vi "Multiple Connections - Server - TCP.vi"() -> ()   [LabVIEW 2011]
doc: "Demonstrates how to establish multiple connections and place them in a queue to be serviced. As connections are made, it sends the current date and time via TCP to all Client VIs that connect to it.\n\nThis VI has two parts -- a loop that listens for each client to connect, and a loop that sends the date and time to each connection in the queue.\n\n<B>Note:</B> Use this VI with Multiple Connections - Client 1.vi and Multiple Connections - Client 2.vi."
panel:
  out "Internal":i32
  out "External":i32
  in  "Port 1":u16=6341
  in  "Port 2":u16=6342
  out "#2 Connections":i32
  out "#1 Connections":i32
  in  "stop":bool
  # "Internal Network"
  # "External Network"
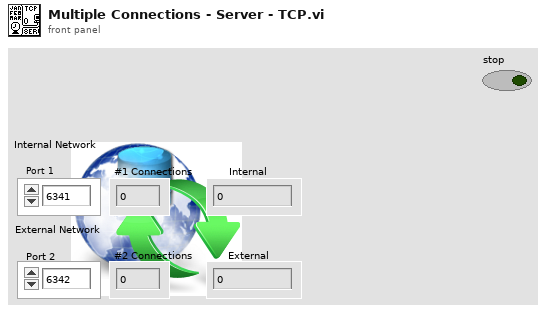
[diagram p1: front panel]
types:
  T1 = enum16{"Obtain", "Enqueue", "Dequeue", "Release"}
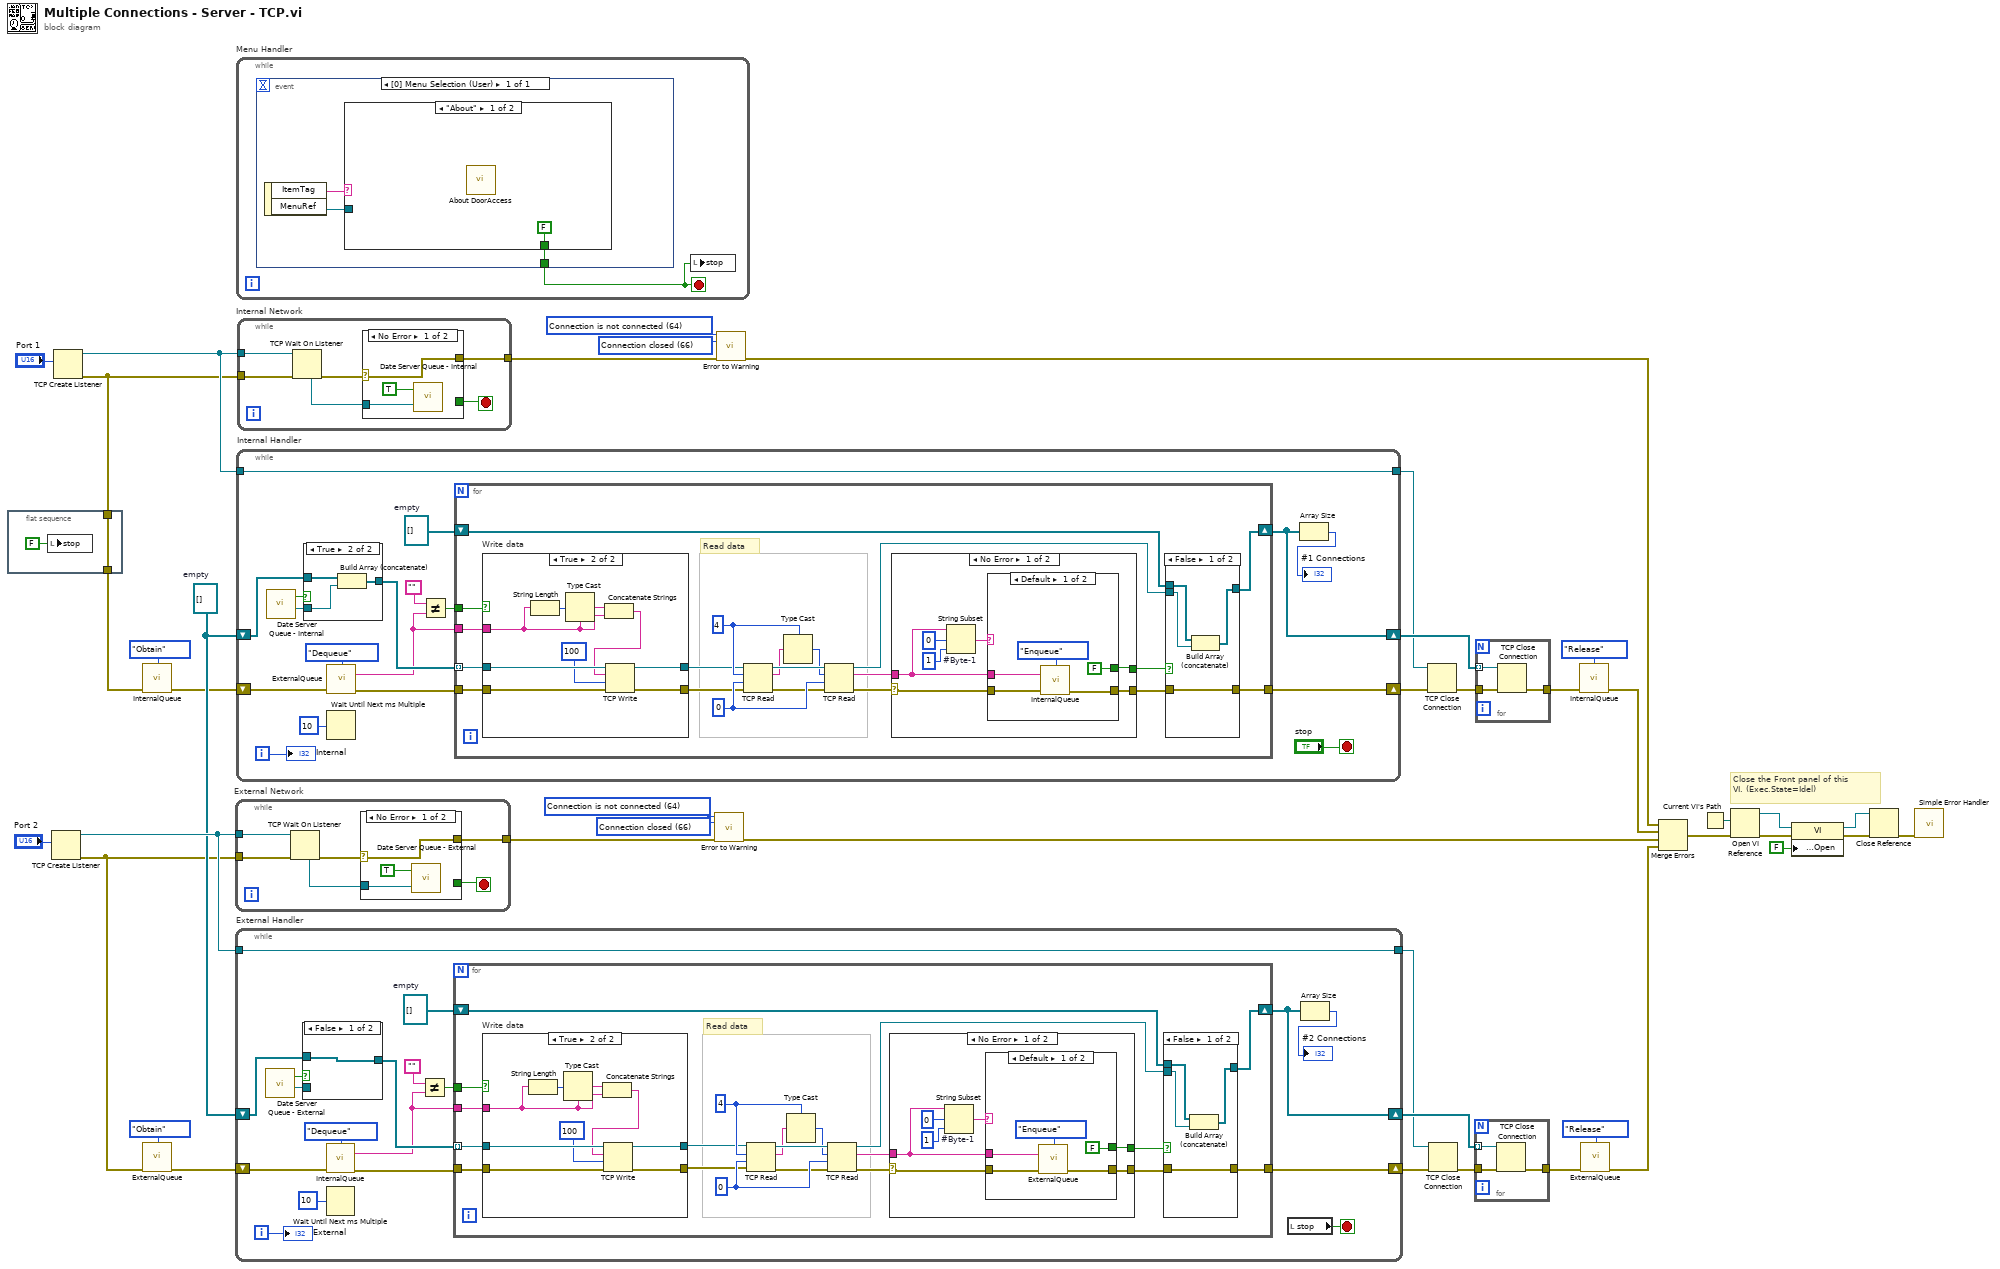
[diagram p0: block diagram]
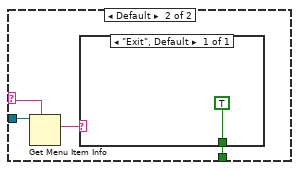
[diagram p2: hidden frame]
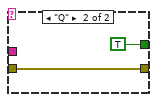
[diagram p3: hidden frame]
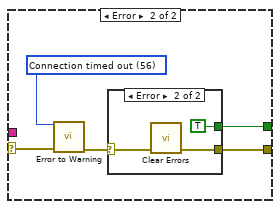
[diagram p4: hidden frame]
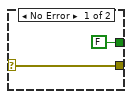
[diagram p5: hidden frame]
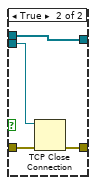
[diagram p7: hidden frame]
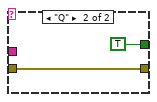
[diagram p9: hidden frame]
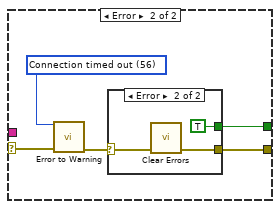
[diagram p10: hidden frame]
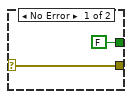
[diagram p11: hidden frame]
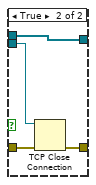
[diagram p13: hidden frame]
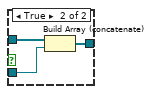
[diagram p14: hidden frame]
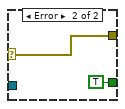
[diagram p15: hidden frame]
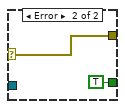
[diagram p16: hidden frame]
diagram:
  w31 = 66 items=["No Error", "Argument Error", "Memory Full", "Out of Zone", "End of File", "File Already Open", "Generic File IO Error", "File Not Found", "File Permission Error", "Disk Full", "Duplicate Path", "Too Many Files Open", "Not Enabled", "Resource File Not Found", "Cannot Add Resource", "Resource Not Found", "Image Not Found", "Image Memory Error", "Pen Does Not Exist", "Config Bad Type", "Config Token Not Found", "Config Parse Error", "Config Memory Error", "Bad External Code Format", "Bad External Code Offset", "External Code Not Present", "Null Window", "Destroy Window Mixup", "Null Menu", "Print Aborted", "Bad Print Record", "Print Driver Error", "Windows Error During Print", "Memory Error During Print", "Print Dialog Error", "Generic Print Error", "Invalid Device Refnum", "Device Not Found", "Device Parameter Error", "Device Unit Error", "Can't Open Device", "Device Call Aborted", "Generic Error", "Cancelled By User", "Object ID Too Low", "Object ID Too High", "Object Not In Heap", "Unknown Heap", "Bad DefProc ID", "DefProc Not In Table", "Message Out Of Range", "Null Method", "Unknown Message", "Manager Call Not Supported", "Bad address", "Connection In progress", "Connection timed out", "Connection is already in progress", "Network attribute not supported", "Network error", "Address in use", "System out of memory", "Connection aborted", "Connection refused", "Connection is not connected", "Connection is already connected", "Connection closed", "Initialize error (interapplication manager)", "Bad occurrence", "Wait on unbound occurrence handler", "Occurrence queue overflow", "Bad path", "Semaphore not signaled", "Unrecognized type (interapplication manager)"] ("2nd Error to Convert")
  w30 = 64 items=["No Error", "Argument Error", "Memory Full", "Out of Zone", "End of File", "File Already Open", "Generic File IO Error", "File Not Found", "File Permission Error", "Disk Full", "Duplicate Path", "Too Many Files Open", "Not Enabled", "Resource File Not Found", "Cannot Add Resource", "Resource Not Found", "Image Not Found", "Image Memory Error", "Pen Does Not Exist", "Config Bad Type", "Config Token Not Found", "Config Parse Error", "Config Memory Error", "Bad External Code Format", "Bad External Code Offset", "External Code Not Present", "Null Window", "Destroy Window Mixup", "Null Menu", "Print Aborted", "Bad Print Record", "Print Driver Error", "Windows Error During Print", "Memory Error During Print", "Print Dialog Error", "Generic Print Error", "Invalid Device Refnum", "Device Not Found", "Device Parameter Error", "Device Unit Error", "Can't Open Device", "Device Call Aborted", "Generic Error", "Cancelled By User", "Object ID Too Low", "Object ID Too High", "Object Not In Heap", "Unknown Heap", "Bad DefProc ID", "DefProc Not In Table", "Message Out Of Range", "Null Method", "Unknown Message", "Manager Call Not Supported", "Bad address", "Connection In progress", "Connection timed out", "Connection is already in progress", "Network attribute not supported", "Network error", "Address in use", "System out of memory", "Connection aborted", "Connection refused", "Connection is not connected", "Connection is already connected", "Connection closed", "Initialize error (interapplication manager)", "Bad occurrence", "Wait on unbound occurrence handler", "Occurrence queue overflow", "Bad path", "Semaphore not signaled", "Unrecognized type (interapplication manager)"] ("1st Error to Convert")
  w15 = refnum<k5>[] []  # empty
  w40 = 66 items=["No Error", "Argument Error", "Memory Full", "Out of Zone", "End of File", "File Already Open", "Generic File IO Error", "File Not Found", "File Permission Error", "Disk Full", "Duplicate Path", "Too Many Files Open", "Not Enabled", "Resource File Not Found", "Cannot Add Resource", "Resource Not Found", "Image Not Found", "Image Memory Error", "Pen Does Not Exist", "Config Bad Type", "Config Token Not Found", "Config Parse Error", "Config Memory Error", "Bad External Code Format", "Bad External Code Offset", "External Code Not Present", "Null Window", "Destroy Window Mixup", "Null Menu", "Print Aborted", "Bad Print Record", "Print Driver Error", "Windows Error During Print", "Memory Error During Print", "Print Dialog Error", "Generic Print Error", "Invalid Device Refnum", "Device Not Found", "Device Parameter Error", "Device Unit Error", "Can't Open Device", "Device Call Aborted", "Generic Error", "Cancelled By User", "Object ID Too Low", "Object ID Too High", "Object Not In Heap", "Unknown Heap", "Bad DefProc ID", "DefProc Not In Table", "Message Out Of Range", "Null Method", "Unknown Message", "Manager Call Not Supported", "Bad address", "Connection In progress", "Connection timed out", "Connection is already in progress", "Network attribute not supported", "Network error", "Address in use", "System out of memory", "Connection aborted", "Connection refused", "Connection is not connected", "Connection is already connected", "Connection closed", "Initialize error (interapplication manager)", "Bad occurrence", "Wait on unbound occurrence handler", "Occurrence queue overflow", "Bad path", "Semaphore not signaled", "Unrecognized type (interapplication manager)"] ("2nd Error to Convert")
  w41 = 64 items=["No Error", "Argument Error", "Memory Full", "Out of Zone", "End of File", "File Already Open", "Generic File IO Error", "File Not Found", "File Permission Error", "Disk Full", "Duplicate Path", "Too Many Files Open", "Not Enabled", "Resource File Not Found", "Cannot Add Resource", "Resource Not Found", "Image Not Found", "Image Memory Error", "Pen Does Not Exist", "Config Bad Type", "Config Token Not Found", "Config Parse Error", "Config Memory Error", "Bad External Code Format", "Bad External Code Offset", "External Code Not Present", "Null Window", "Destroy Window Mixup", "Null Menu", "Print Aborted", "Bad Print Record", "Print Driver Error", "Windows Error During Print", "Memory Error During Print", "Print Dialog Error", "Generic Print Error", "Invalid Device Refnum", "Device Not Found", "Device Parameter Error", "Device Unit Error", "Can't Open Device", "Device Call Aborted", "Generic Error", "Cancelled By User", "Object ID Too Low", "Object ID Too High", "Object Not In Heap", "Unknown Heap", "Bad DefProc ID", "DefProc Not In Table", "Message Out Of Range", "Null Method", "Unknown Message", "Manager Call Not Supported", "Bad address", "Connection In progress", "Connection timed out", "Connection is already in progress", "Network attribute not supported", "Network error", "Address in use", "System out of memory", "Connection aborted", "Connection refused", "Connection is not connected", "Connection is already connected", "Connection closed", "Initialize error (interapplication manager)", "Bad occurrence", "Wait on unbound occurrence handler", "Occurrence queue overflow", "Bad path", "Semaphore not signaled", "Unrecognized type (interapplication manager)"] ("1st Error to Convert")
  # "Close the Front panel of this\nVI. (Exec.State=Idel)"
  n1 = flat-sequence {
    tunnel: [w43] -> w5
    tunnel: w4 -> [w43]
    frame #0 {
      n2 = local write "stop"(FALSE ("stop")) -> ()
    }
  }
  n3 = TCP Create Listener(10:"Port 2") -> (0:w12:errorcluster, 3:w28:refnum<k5>)  [unwired: 1 in, 4 out]
  n4 = TCP Create Listener(10:"Port 1") -> (0:w4:errorcluster, 3:w16:refnum<k5>)  [unwired: 1 in, 4 out]
  n5 = call "InternalQueue.vi"("Mode"=T1."Obtain", "error in (no error)"=w5) -> ("error out"=w14:errorcluster)  [unwired: 12 in, 1 out]
  n6 = call "ExternalQueue.vi"("Mode"=T1."Obtain", "error in (no error)"=w12) -> ("error out"=w13:errorcluster)  [unwired: 12 in, 1 out]
  n7 = while "External Network" {
    tunnel: w28 -> [w49]
    tunnel: w12 -> [w50]
    tunnel: [w45] -> w29
    stop <- w46 stop-if-true
    n8 = TCP Wait On Listener(8:w50, 11:w49) -> (0:w47:errorcluster, 4:w48:refnum<k5>)  [unwired: 5 out]
    n9 = case shown="No Error" w47 {
      selector: w47 -> [w51 w54]
      tunnel: w48 -> [w52 _]
      tunnel: [_ TRUE] -> w46
      tunnel: [w51 w54] -> w45
      frame No Error {
        n10 = call "Date Server Queue - External.vi"("new value"=w52, "set queue? (F: de-queue)"=TRUE) -> ()  [unwired: 2 out]
      }
      frame Error {
      }
    }
  }
  n11 = while "External Handler" {
    shift-left: w15 -> [w71]
    shift-right: [w68] -> w27
    tunnel: w28 -> [w67]
    tunnel: [w67] -> w2
    shift-right: [w66] -> w34
    shift-left: w13 -> [w64]
    i -> [w56]
    stop <- w62 stop-if-true
    w69 = refnum<k5>[] []  # empty
    n12 = call "Date Server Queue - External.vi"() -> ("value"=w73:refnum<k5>, "valid?"=w72:bool)  [unwired: 2 in]
    n13 = case shown="False" w72 {
      tunnel: w73 -> [_ w140]
      tunnel: w71 -> [w137 w139]
      tunnel: [w137 w138] -> w70
      frame False {
      }
      frame True {
        n14 = Build Array (concatenate)(w139, w140) -> (w138:refnum<k5>[])
      }
    }
    n15 = call "InternalQueue.vi"("Mode"=T1."Dequeue", "error in (no error)"=w64) -> ("Queue Out"=w59:string, "error out"=w63:errorcluster)  [unwired: 12 in]
    n16 = Wait Until Next ms Multiple(millisecond multiple=u32 10) -> ()  [unwired: 1 out]
    n17 = Not Equal?(x="", y=w59) -> (x != y?=w58:bool)
    n18 = for {
      tunnel: w70 -> [w90] mode=indexing
      shift-right: [w91] -> w68
      shift-left: w69 -> [w93]
      tunnel: [w92] -> w66
      tunnel: w63 -> [w89]
      tunnel: w59 -> [w86]
      tunnel: w58 -> [w85]
      w84 = 0 ("timeout ms (25000)")
      w82 = 4
      # "Read data"
      n19 = case "Write data" shown="True" w85 {
        tunnel: w90 -> [w119 w124]
        tunnel: w89 -> [w118 w126]
        tunnel: [w118 w122] -> w74
        tunnel: w86 -> [_ w125]
        tunnel: [w119 w120] -> w75
        frame False {
        }
        frame True {
          n20 = String Length(string=w125) -> (length=w128:i32)
          n21 = Type Cast(type=w125, x=w128) -> (*(type *) &x=w127:string)
          n22 = Concatenate Strings(w127, w125) -> (w121:string)
          n23 = TCP Write(connection ID=w124, data in=w121, error in (no error)=w126, 9:100 ("timeout ms (25000)")) -> (connection ID out=w120:refnum<k5>, error out=w122:errorcluster)  [unwired: 1 out]
        }
      }
      n24 = TCP Read(connection ID=w75, bytes to read=w82, error in (no error)=w74, 9:w84) -> (connection ID out=w83:refnum<k5>, data out=w81:string, error out=w80:errorcluster)  [unwired: 1 out]
      n25 = Type Cast(type=w82, x=w81) -> (*(type *) &x=w79:i32)
      n26 = TCP Read(connection ID=w83, bytes to read=w79, error in (no error)=w80, 9:w84) -> (connection ID out=w78:refnum<k5>, data out=w77:string, error out=w76:errorcluster)  [unwired: 1 out]
      n27 = case shown="No Error" w76 {
        selector: w76 -> [w96 w112]
        tunnel: [w95 w109] -> w87
        tunnel: [w94 w108] -> w88
        tunnel: w77 -> [w97 _]
        frame No Error {
          n28 = String Subset "#Byte-1"(string=w97, offset (0)=0, length (rest)=1 ("length (rest)")) -> (substring=w98:string)
          n29 = case shown="Default" w98 {
            tunnel: w97 -> [w101 _]
            tunnel: w96 -> [w103 w107]
            tunnel: [w102 w107] -> w95
            tunnel: [FALSE TRUE] -> w94
            frame Default {
              n30 = call "ExternalQueue.vi"("Mode"=T1."Enqueue", "Queue In"=w101, "error in (no error)"=w103) -> ("error out"=w102:errorcluster)  [unwired: 11 in, 1 out]
            }
            frame "Q" {
            }
          }
        }
        frame Error {
          w111 = 56 items=["No Error", "Argument Error", "Memory Full", "Out of Zone", "End of File", "File Already Open", "Generic File IO Error", "File Not Found", "File Permission Error", "Disk Full", "Duplicate Path", "Too Many Files Open", "Not Enabled", "Resource File Not Found", "Cannot Add Resource", "Resource Not Found", "Image Not Found", "Image Memory Error", "Pen Does Not Exist", "Config Bad Type", "Config Token Not Found", "Config Parse Error", "Config Memory Error", "Bad External Code Format", "Bad External Code Offset", "External Code Not Present", "Null Window", "Destroy Window Mixup", "Null Menu", "Print Aborted", "Bad Print Record", "Print Driver Error", "Windows Error During Print", "Memory Error During Print", "Print Dialog Error", "Generic Print Error", "Invalid Device Refnum", "Device Not Found", "Device Parameter Error", "Device Unit Error", "Can't Open Device", "Device Call Aborted", "Generic Error", "Cancelled By User", "Object ID Too Low", "Object ID Too High", "Object Not In Heap", "Unknown Heap", "Bad DefProc ID", "DefProc Not In Table", "Message Out Of Range", "Null Method", "Unknown Message", "Manager Call Not Supported", "Bad address", "Connection In progress", "Connection timed out", "Connection is already in progress", "Network attribute not supported", "Network error", "Address in use", "System out of memory", "Connection aborted", "Connection refused", "Connection is not connected", "Connection is already connected", "Connection closed", "Initialize error (interapplication manager)", "Bad occurrence", "Wait on unbound occurrence handler", "Occurrence queue overflow", "Bad path", "Semaphore not signaled", "Unrecognized type (interapplication manager)"] ("1st Error to Convert")
          n31 = call <vilib>:"Error to Warning.vi"("1st Error to Convert"=w111, "error in"=w112) -> ("warning out"=w110:errorcluster)  [unwired: 13 in]
          n32 = case shown="Error" w110 {
            selector: w110 -> [w114 w117]
            tunnel: [w114 w116] -> w109
            tunnel: [FALSE TRUE] -> w108
            frame No Error {
            }
            frame Error {
              n33 = call <vilib>:"Clear Errors.vi"("error in (no error)"=w117) -> ("error out"=w116:errorcluster)  [unwired: 6 in]
            }
          }
        }
      }
      n34 = case shown="False" w88 {
        tunnel: w93 -> [w132 w136]
        tunnel: w78 -> [w131 w135]
        tunnel: [w130 w136] -> w91
        tunnel: w87 -> [w129 w134]
        tunnel: [w129 w133] -> w92
        frame False {
          n35 = Build Array (concatenate)(w132, w131) -> (w130:refnum<k5>[])
        }
        frame True {
          n36 = TCP Close Connection(connection ID=w135, error in (no error)=w134) -> (error out=w133:errorcluster)  [unwired: 2 out]
        }
      }
    }
    n37 = local read "stop"() -> (w62:bool)
    n38 = Array Size(array=w68) -> (size(s)=→"#2 Connections":i32)
    "External" <- w56
  }
  n39 = while "Menu Handler" {
    stop <- w141 stop-if-true
    n40 = event shown="[0] Menu Selection (User)" {
      selector: _ -> [_]
      dyn-events: _ -> [_]
      timeout: _ -> [_]
      tunnel: [w142] -> w141
      event Menu Selection (User) {
        n41 = event-data() -> ("ItemTag"=w143:string, "MenuRef"=w144:refnum<k9>)  [unwired: 1 in]
        n42 = case shown="\"About\"" w143 {
          selector: w143 -> [_ w148]
          tunnel: w144 -> [_ w149]
          tunnel: [FALSE w146] -> w142
          frame "About" {
            n43 = call "About DoorAccess.vi"() -> ()  [unwired: 1 out]
          }
          frame Default {
            n44 = Get Menu Item Info(7:w148, 11:w149) -> (2:w147:string)  [unwired: 1 in, 6 out]
            n45 = case shown="\"Exit\", Default" w147 {
              tunnel: [TRUE] -> w146
              frame "Exit", Default {
              }
            }
          }
        }
      }
    }
    n46 = local write "stop"(w141) -> ()
  }
  n47 = while "Internal Handler" {
    shift-left: w15 -> [w166]
    shift-right: [w163] -> w17
    tunnel: w16 -> [w162]
    tunnel: [w162] -> w1
    shift-right: [w161] -> w18
    shift-left: w14 -> [w159]
    i -> [w151]
    stop <- "stop" stop-if-true
    w164 = refnum<k5>[] []  # empty
    n48 = call "Date Server Queue - Internal.vi"() -> ("value"=w168:refnum<k5>, "valid?"=w167:bool)  [unwired: 2 in]
    n49 = case shown="True" w167 {
      tunnel: w168 -> [_ w235]
      tunnel: w166 -> [w232 w234]
      tunnel: [w232 w233] -> w165
      frame False {
      }
      frame True {
        n50 = Build Array (concatenate)(w234, w235) -> (w233:refnum<k5>[])
      }
    }
    n51 = call "ExternalQueue.vi"("Mode"=T1."Dequeue", "error in (no error)"=w159) -> ("Queue Out"=w155:string, "error out"=w158:errorcluster)  [unwired: 12 in]
    n52 = Wait Until Next ms Multiple(millisecond multiple=u32 10) -> ()  [unwired: 1 out]
    n53 = Not Equal?(x="", y=w155) -> (x != y?=w154:bool)
    n54 = for {
      tunnel: w165 -> [w185] mode=indexing
      shift-right: [w186] -> w163
      shift-left: w164 -> [w188]
      tunnel: [w187] -> w161
      tunnel: w158 -> [w184]
      tunnel: w155 -> [w181]
      tunnel: w154 -> [w180]
      w179 = 0 ("timeout ms (25000)")
      w177 = 4
      # "Read data"
      n55 = case "Write data" shown="True" w180 {
        tunnel: w185 -> [w214 w219]
        tunnel: w184 -> [w213 w221]
        tunnel: [w213 w217] -> w173
        tunnel: w181 -> [_ w220]
        tunnel: [w214 w215] -> w172
        frame False {
        }
        frame True {
          n56 = String Length(string=w220) -> (length=w223:i32)
          n57 = Type Cast(type=w220, x=w223) -> (*(type *) &x=w222:string)
          n58 = Concatenate Strings(w222, w220) -> (w216:string)
          n59 = TCP Write(connection ID=w219, data in=w216, error in (no error)=w221, 9:100 ("timeout ms (25000)")) -> (connection ID out=w215:refnum<k5>, error out=w217:errorcluster)  [unwired: 1 out]
        }
      }
      n60 = TCP Read(connection ID=w172, bytes to read=w177, error in (no error)=w173, 9:w179) -> (connection ID out=w178:refnum<k5>, data out=w176:string, error out=w175:errorcluster)  [unwired: 1 out]
      n61 = Type Cast(type=w177, x=w176) -> (*(type *) &x=w174:i32)
      n62 = TCP Read(connection ID=w178, bytes to read=w174, error in (no error)=w175, 9:w179) -> (connection ID out=w171:refnum<k5>, data out=w169:string, error out=w170:errorcluster)  [unwired: 1 out]
      n63 = case shown="No Error" w170 {
        selector: w170 -> [w191 w207]
        tunnel: [w190 w204] -> w182
        tunnel: [w189 w203] -> w183
        tunnel: w169 -> [w192 _]
        frame No Error {
          n64 = String Subset "#Byte-1"(string=w192, offset (0)=0, length (rest)=1 ("length (rest)")) -> (substring=w193:string)
          n65 = case shown="Default" w193 {
            tunnel: w192 -> [w196 _]
            tunnel: w191 -> [w198 w202]
            tunnel: [w197 w202] -> w190
            tunnel: [FALSE TRUE] -> w189
            frame Default {
              n66 = call "InternalQueue.vi"("Mode"=T1."Enqueue", "Queue In"=w196, "error in (no error)"=w198) -> ("error out"=w197:errorcluster)  [unwired: 11 in, 1 out]
            }
            frame "Q" {
            }
          }
        }
        frame Error {
          w206 = 56 items=["No Error", "Argument Error", "Memory Full", "Out of Zone", "End of File", "File Already Open", "Generic File IO Error", "File Not Found", "File Permission Error", "Disk Full", "Duplicate Path", "Too Many Files Open", "Not Enabled", "Resource File Not Found", "Cannot Add Resource", "Resource Not Found", "Image Not Found", "Image Memory Error", "Pen Does Not Exist", "Config Bad Type", "Config Token Not Found", "Config Parse Error", "Config Memory Error", "Bad External Code Format", "Bad External Code Offset", "External Code Not Present", "Null Window", "Destroy Window Mixup", "Null Menu", "Print Aborted", "Bad Print Record", "Print Driver Error", "Windows Error During Print", "Memory Error During Print", "Print Dialog Error", "Generic Print Error", "Invalid Device Refnum", "Device Not Found", "Device Parameter Error", "Device Unit Error", "Can't Open Device", "Device Call Aborted", "Generic Error", "Cancelled By User", "Object ID Too Low", "Object ID Too High", "Object Not In Heap", "Unknown Heap", "Bad DefProc ID", "DefProc Not In Table", "Message Out Of Range", "Null Method", "Unknown Message", "Manager Call Not Supported", "Bad address", "Connection In progress", "Connection timed out", "Connection is already in progress", "Network attribute not supported", "Network error", "Address in use", "System out of memory", "Connection aborted", "Connection refused", "Connection is not connected", "Connection is already connected", "Connection closed", "Initialize error (interapplication manager)", "Bad occurrence", "Wait on unbound occurrence handler", "Occurrence queue overflow", "Bad path", "Semaphore not signaled", "Unrecognized type (interapplication manager)"] ("1st Error to Convert")
          n67 = call <vilib>:"Error to Warning.vi"("1st Error to Convert"=w206, "error in"=w207) -> ("warning out"=w205:errorcluster)  [unwired: 13 in]
          n68 = case shown="Error" w205 {
            selector: w205 -> [w209 w212]
            tunnel: [w209 w211] -> w204
            tunnel: [FALSE TRUE] -> w203
            frame No Error {
            }
            frame Error {
              n69 = call <vilib>:"Clear Errors.vi"("error in (no error)"=w212) -> ("error out"=w211:errorcluster)  [unwired: 6 in]
            }
          }
        }
      }
      n70 = case shown="False" w183 {
        tunnel: w188 -> [w227 w231]
        tunnel: w171 -> [w226 w230]
        tunnel: [w225 w231] -> w186
        tunnel: w182 -> [w224 w229]
        tunnel: [w224 w228] -> w187
        frame False {
          n71 = Build Array (concatenate)(w227, w226) -> (w225:refnum<k5>[])
        }
        frame True {
          n72 = TCP Close Connection(connection ID=w230, error in (no error)=w229) -> (error out=w228:errorcluster)  [unwired: 2 out]
        }
      }
    }
    n73 = Array Size(array=w163) -> (size(s)=→"#1 Connections":i32)
    "Internal" <- w151
  }
  n74 = while "Internal Network" {
    tunnel: w16 -> [w240]
    tunnel: w4 -> [w241]
    tunnel: [w236] -> w42
    stop <- w237 stop-if-true
    n75 = TCP Wait On Listener(8:w241, 11:w240) -> (0:w238:errorcluster, 4:w239:refnum<k5>)  [unwired: 5 out]
    n76 = case shown="No Error" w238 {
      selector: w238 -> [w242 w245]
      tunnel: w239 -> [w243 _]
      tunnel: [_ TRUE] -> w237
      tunnel: [w242 w245] -> w236
      frame No Error {
        n77 = call "Date Server Queue - Internal.vi"("new value"=w243, "set queue? (F: de-queue)"=TRUE) -> ()  [unwired: 2 out]
      }
      frame Error {
      }
    }
  }
  n78 = call <vilib>:"Error to Warning.vi"("1st Error to Convert"=w30, "2nd Error to Convert"=w31, "error in"=w29) -> ("warning out"=w26:errorcluster)  [unwired: 2 in, 10 out]
  n79 = call <vilib>:"Error to Warning.vi"("1st Error to Convert"=w41, "2nd Error to Convert"=w40, "error in"=w42) -> ("warning out"=w37:errorcluster)  [unwired: 2 in, 10 out]
  n80 = TCP Close Connection(connection ID=w1, error in (no error)=w18) -> (error out=w38:errorcluster)  [unwired: 2 out]
  n81 = TCP Close Connection(connection ID=w2, error in (no error)=w34) -> (error out=w33:errorcluster)  [unwired: 2 out]
  n82 = for {
    tunnel: w27 -> [w249] mode=indexing
    tunnel: [w248] -> w8
    tunnel: w33 -> [w247]
    n83 = TCP Close Connection(connection ID=w249, error in (no error)=w247) -> (error out=w248:errorcluster)  [unwired: 2 out]
  }
  n84 = for {
    tunnel: w17 -> [w252] mode=indexing
    tunnel: [w251] -> w10
    tunnel: w38 -> [w250]
    n85 = TCP Close Connection(connection ID=w252, error in (no error)=w250) -> (error out=w251:errorcluster)  [unwired: 2 out]
  }
  n86 = call "InternalQueue.vi"("Mode"=T1."Release", "error in (no error)"=w10) -> ("error out"=w9:errorcluster)  [unwired: 12 in, 1 out]
  n87 = call "ExternalQueue.vi"("Mode"=T1."Release", "error in (no error)"=w8) -> ("error out"=w7:errorcluster)  [unwired: 12 in, 1 out]
  n88 = Merge Errors(w37, w9, w26, w7) -> (w3:errorcluster)
  n89 = Current VI's Path() -> (path=w25:path)
  n90 = Open VI Reference(vi path=w25, error in (no error)=w3) -> (vi reference=w20:refnum<vi>, error out=w24:errorcluster)  [unwired: 4 in]
  n91 = property class="VI"(reference=w20, error in=w24, "Front Panel Window:Open"=FALSE) -> (reference out=w23:refnum<vi>, error out=w21:errorcluster)
  n92 = Close Reference(reference=w23, error in (no error)=w21) -> (error out=w19:errorcluster)
  n93 = call <vilib>:"Simple Error Handler.vi"("error in (no error)"=w19) -> ()  [unwired: 1 in, 8 out]
